vi "View one AI param.vi"(5 "ActivateAIView":bool, 7 "conninfo":T4={"host"="localhost", "port"="5432", "client_encoding"="WIN1251", "dbname"="system", "user"="postgres", "password"=""}, 9 "AIP":T2, 10 "AI_State":T1[](array[typedef]), 11 "AITable":dbl[](array[numeric]) format="%#.0f") -> (0 "error out":errorcluster)   [LabVIEW 2019, in "Inputs.lvlib"]
uses:
  Inputs.lvlib
  Database/ctl/Coninfo.ctl
  Ctl/AI.ctl
  Ctl/AI short.ctl
  Ctl/Parameter State.ctl
  Ctl/AIParamColumns.ctl
  Database/PostgreSQL2LabVIEW/libpqUtility64/src/PQexecute.vi
  Database/PostgreSQL2LabVIEW/libpqUtility64/src/PQconnect.vi
  Database/PostgreSQL2LabVIEW/libpqUtility64/src/PQclose.vi
  Database/PostgreSQL2LabVIEW/libpqlv64/src/PQresultErrorMessage.vi
  Database/PostgreSQL2LabVIEW/libpqUtility64/src/PQclear.vi
  Database/PostgreSQL2LabVIEW/libpqlv64/src/PQsendQuery.vi
  Database/PostgreSQL2LabVIEW/libpqlv64/src/PQgetResult.vi
  Database/PostgreSQL2LabVIEW/libpqlv64/src/PQresultStatus.vi
  Database/PostgreSQL2LabVIEW/libpqlv64/src/PQfinish.vi
  Database/PostgreSQL2LabVIEW/libpqlv64/src/PQconnectdb.vi
  Database/PostgreSQL2LabVIEW/libpqlv64/src/PQerrorMessage.vi
  Database/PostgreSQL2LabVIEW/libpqlv64/src/PQstatus.vi
  Database/PostgreSQL2LabVIEW/libpqlv64/src/PQclear.vi
  Database/PostgreSQL.lvlib
panel:
  in  "instrument_min_offset":dbl min=-32768.0 max=65535.0 step=1.0 format="%#.0f"
  in  "time_const":dbl min=-32768.0 max=65535.0 step=1.0 format="%#.0f"
  in  "instrument_offset":dbl min=-32768.0 max=65535.0 step=1.0 format="%#.0f"
  in  "instrument_gain":dbl min=-32768.0 max=65535.0 step=1.0 format="%#.0f"
  out "fcode_full":string="кгс/см2"
  out "AI_1":dbl format="%#.1f"
  in  "Param":i32[](listbox) caption="Параметры"
  in  "fcodef":string
  in  "fcode":string
  in  "d":dbl min=-32768.0 max=65535.0 step=1.0 format="%#.0f"
  in  "instrument_max_offset":dbl min=-32768.0 max=65535.0 step=1.0 format="%#.0f"
  in  "input_pv_max":dbl format="%#.1f"
  in  "input_pv_min":dbl format="%#.1f"
  in  "input_register_max":dbl min=-32768.0 max=65535.0 step=1.0 format="%#.0f"
  in  "input_register_min":dbl min=-32768.0 max=65535.0 step=1.0 format="%#.0f"
  out "units":string="кгс/см2"
  in  "instrument_range_max":dbl format="%#.1f"
  in  "process_range_max":dbl format="%#.1f"
  in  "process_high_acd":dbl format="%#.1f"
  in  "process_high_alr":dbl format="%#.1f"
  in  "process_low_alr":dbl format="%#.1f"
  in  "process_low_acd":dbl format="%#.1f"
  in  "process_range_min":dbl format="%#.1f"
  in  "instrument_range_min":dbl format="%#.1f"
  # "Настройка пределов"
  # "верхнийний предел датчика"
  # "верхний предел достоверных показаний"
  # "верхний аварийный предел"
  # "верхний предупредительный предел"
  # "нижний предупредительный предел"
  # "нижний аварийный предел"
  # "нижний предел достоверных показаний"
  # "нижний предел датчика"
  # "Настройка датчика"
  # "Y"
  # "значение сигнала максимум (Ymax)"
  # "значение сигнала минимум (Ymin)"
  # "X"
  # "входной регистр минимум (Xmin)"
  # "входной регистр максимум (Xmax)"
  # "Analog parameters"
  # "Description of analog parameters"
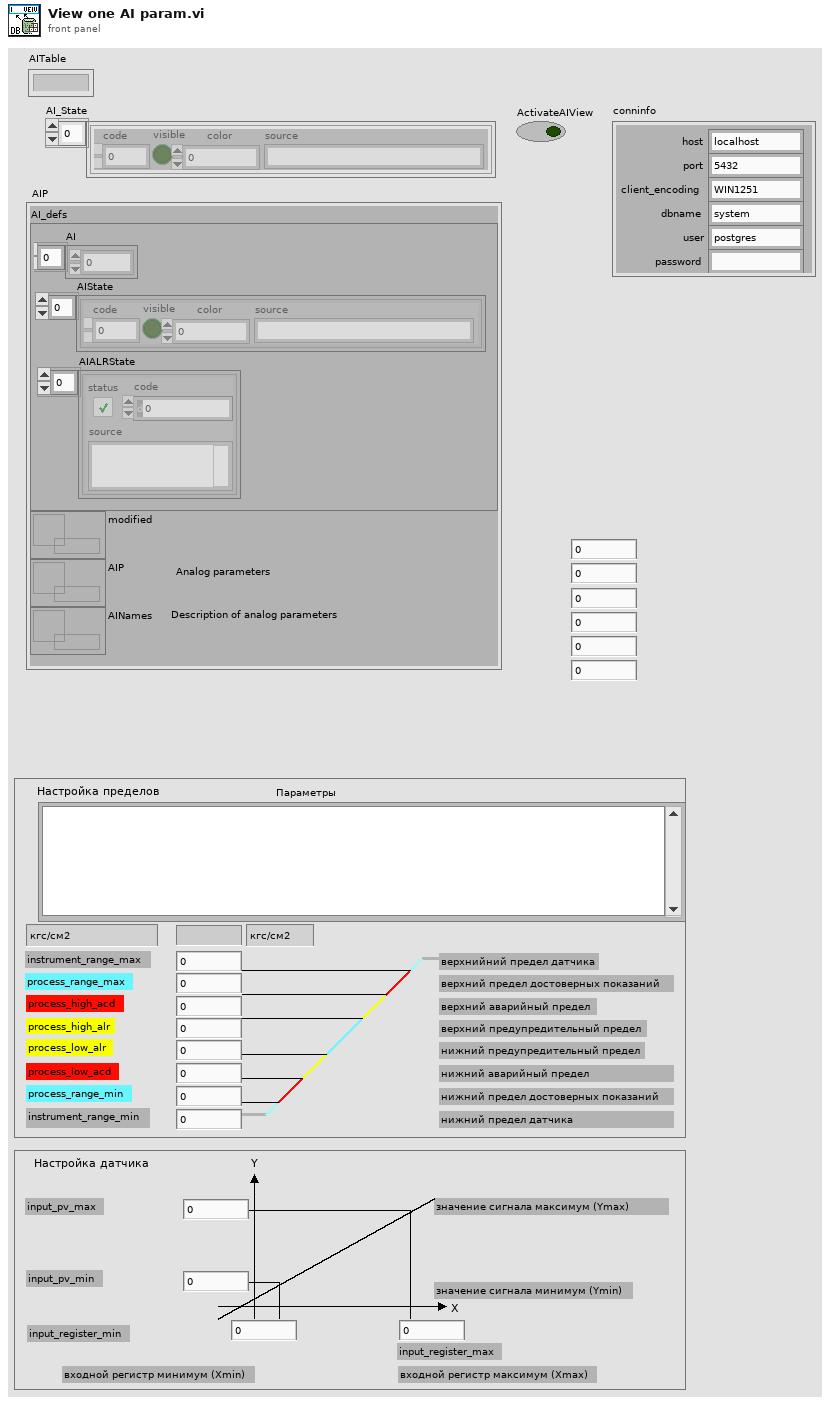
[diagram p1: front panel]
types:
  T1 = typedef "Inputs.lvlib/Parameter State.ctl" = cluster{"code":i32, "visible":bool, "color":u32, "source":string}
  T2 = typedef "Inputs.lvlib/AI.ctl" = cluster{"AI_defs":T3, "modified":refnum<data-value>, "AIP":refnum<data-value>, "AINames":refnum<data-value>}
  T3 = typedef "Inputs.lvlib/AI short.ctl" = cluster{"AI":dbl[], "AIState":T1[], "AIALRState":errorcluster[]}
  T4 = typedef "PostgreSQL.lvlib/Coninfo.ctl" = cluster{"host":string, "port":string, "client_encoding":string, "dbname":string, "user":string, "password":string}
  T5 = enum32{"Invalid", "Standard", "Closed", "Hidden", "Minimized", "Maximized"}
  T6 = typedef "Inputs.lvlib/AIParamColumns.ctl" = enum16{"instrument_gain", "instrument_offset", "time_const", "instrument_min_offset", "instrument_range_min", "process_range_min", "process_low_acd", "process_low_alr", "process_high_alr", "process_high_acd", "process_range_max", "instrument_range_max", "instrument_max_offset", "d", "input_register_min", "input_register_max", "input_pv_min", "input_pv_max", "module_fcode_full", "control_channel_num", "ip_adress", "fcode", "fcodef", "fcode_full", "fname", "process_units"}
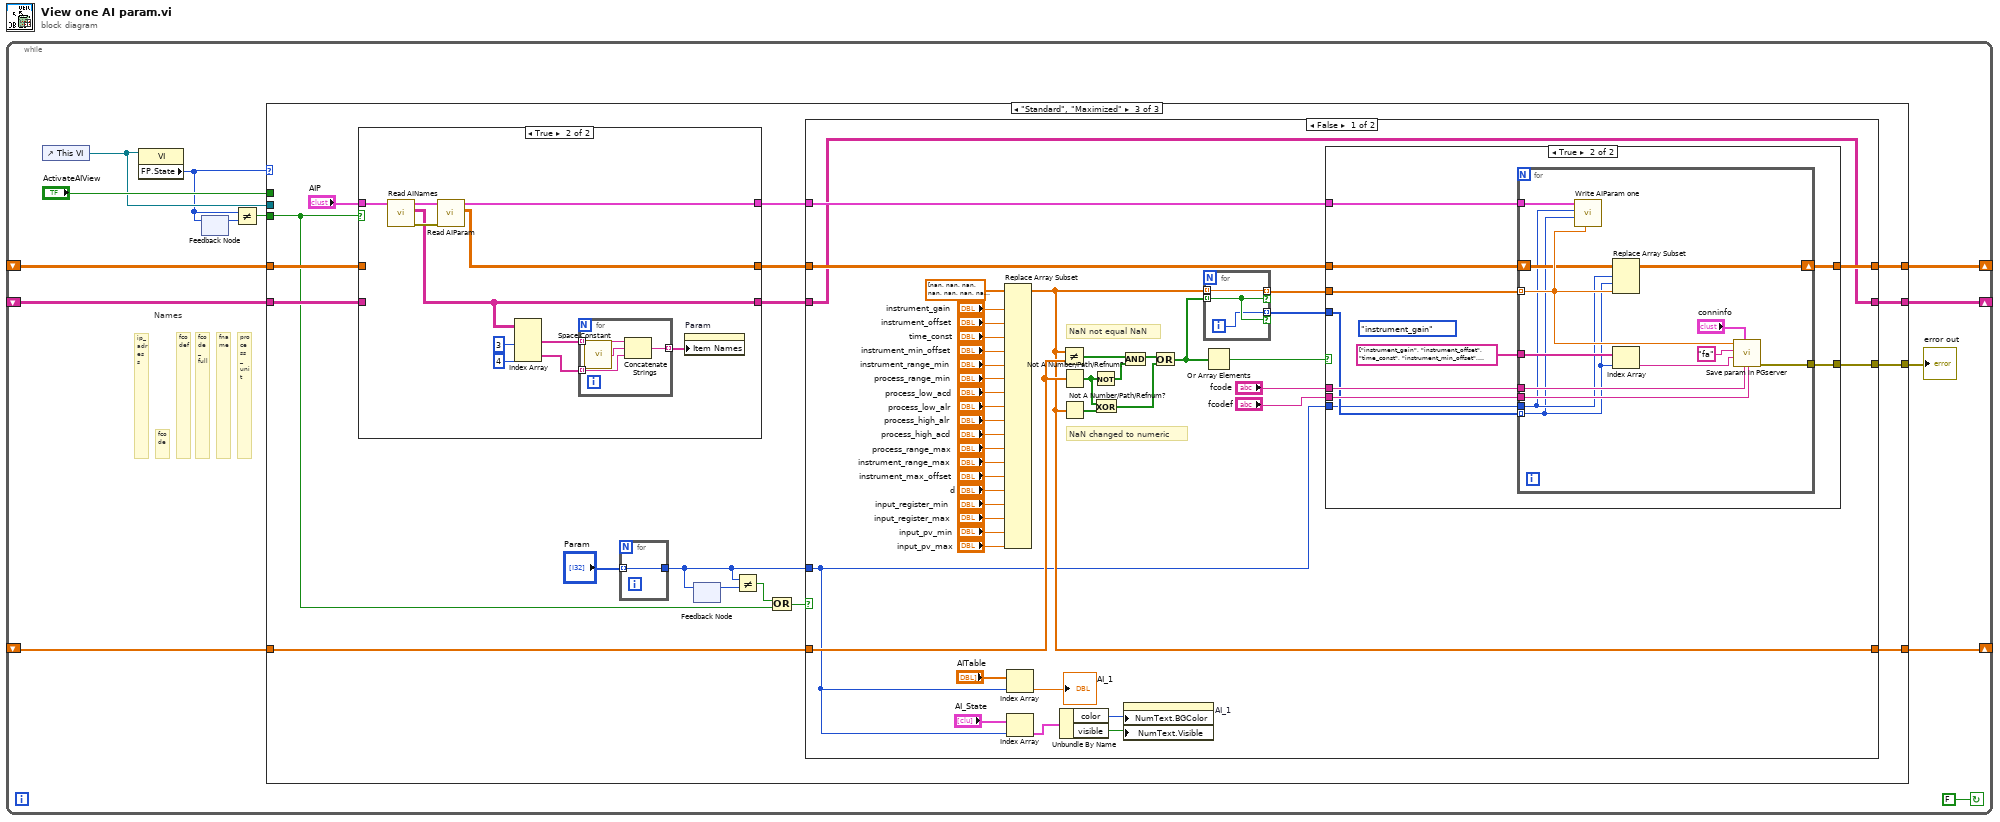
[diagram p0: block diagram]
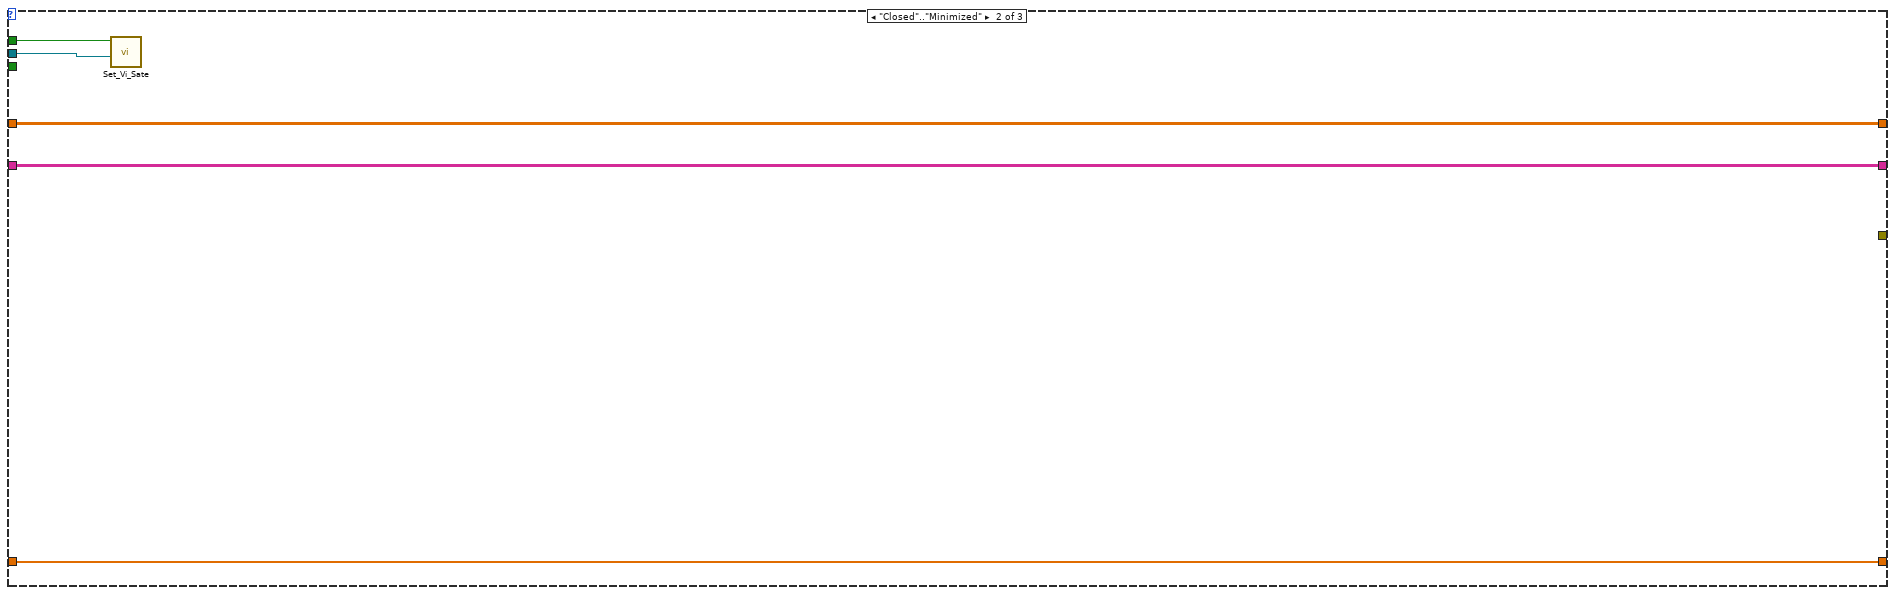
[diagram p3: hidden frame]
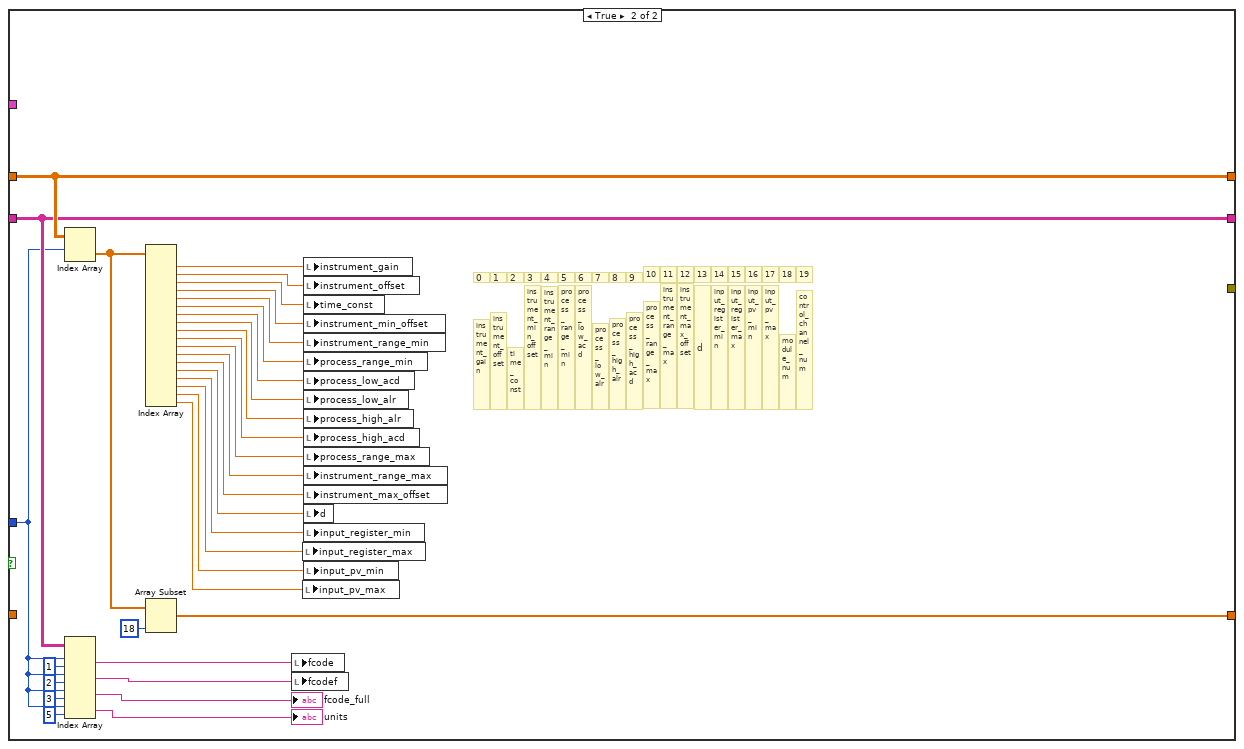
[diagram p6: hidden frame]
diagram:
  n1 = while {
    shift-right: [w6] -> _
    shift-left: _ -> [w4]
    shift-right: [w5] -> _
    shift-left: _ -> [w3]
    shift-right: [w2] -> _
    shift-left: _ -> [w1]
    stop <- FALSE continue-if-true
    # "fcodef"
    # "ip_adress"
    # "process_unit"
    # "fname"
    # "fcode_full"
    # "fcode"
    # "Names"
    n2 = control-ref of="This VI"() -> (w12:refnum<vi>)
    n3 = property class="VI"(reference=w12) -> ("FP.State"=w9:T5)  [unwired: 1 in, 2 out]
    n4 = feedback #1() -> (w10:T5)  [unwired: 1 in]
    n5 = feedback-in #1(w9) -> ()
    n6 = Not Equal?(x=w9, y=w10) -> (x != y?=w8:bool)
    n7 = case shown="\"Standard\", \"Maximized\"" w9 {
      tunnel: "ActivateAIView" -> [_ w21 _]
      tunnel: w12 -> [_ w20 _]
      tunnel: [_ _ w28] -> w11
      tunnel: w8 -> [_ _ w30]
      tunnel: [w16 w19 w22] -> w6
      tunnel: [w15 w18 w24] -> w5
      tunnel: w4 -> [w16 w19 w32]
      tunnel: w3 -> [w15 w18 w31]
      tunnel: [w14 w17 w27] -> w2
      tunnel: w1 -> [w14 w17 w26]
      frame "Invalid", Default {
      }
      frame "Closed".."Minimized" {
        n8 = call "Set_Vi_Sate.vi"("VI"=w20, "Activate (F)"=w21) -> ()  [unwired: 9 in, 1 out]
      }
      frame "Standard", "Maximized" {
        n9 = case shown="True" w30 {
          tunnel: [w41 w45] -> w25
          tunnel: [w42 w44] -> w33
          tunnel: "AIP" -> [w40 w46]
          tunnel: w32 -> [w42 _]
          tunnel: w31 -> [w41 _]
          tunnel: [w40 w43] -> w23
          frame False {
          }
          frame True {
            n10 = call "Read AINames.vi"("AI in"=w46) -> ("error out"=w48:errorcluster, "AINames"=w45:string[][], "AI out"=w47:T2)  [unwired: 8 in]
            n11 = call "Read AIParam.vi"("error in (no error)"=w48, "AI in"=w47) -> ("AIParam"=w44:dbl[][], "AI out"=w43:T2)  [unwired: 7 in, 1 out]
            n12 = Index Array(array=w45, index (col) #1=3 ("index (row)"), index (col) #2=4 ("index (row)")) -> (element #1=w52:string[], element #2=w50:string[])  [unwired: 2 in]
            n13 = for {
              tunnel: w52 -> [w57] mode=indexing
              tunnel: w50 -> [w55] mode=indexing
              tunnel: [w54] -> w49 mode=indexing
              n14 = call <vilib>:"Space Constant.vi"() -> ("String"=w56:string)
              n15 = Concatenate Strings(w57, w56, w55) -> (w54:string)
            }
            n16 = property on="Param" class="LstBox (strict)"("Item Names"=w49) -> ()  [unwired: 2 in, 2 out]
          }
        }
        n17 = for {
          tunnel: "Param" -> [w39] mode=indexing
          tunnel: [w39] -> w29
        }
        n18 = feedback #2() -> (w38:i32)  [unwired: 1 in]
        n19 = feedback-in #2(w29) -> ()
        n20 = Not Equal?(x=w29, y=w38) -> (x != y?=w36:bool)
        n21 = Or(x=w36, y=w30) -> (x .or. y?=w37:bool)
        n22 = case shown="False" w37 {
          tunnel: w29 -> [w63 w136]
          tunnel: w25 -> [w64 w141]
          tunnel: w33 -> [w82 w142]
          tunnel: [w85 _] -> w28
          tunnel: [w70 w140] -> w27
          tunnel: w26 -> [w73 _]
          tunnel: [w74 w142] -> w22
          tunnel: [w64 w141] -> w24
          tunnel: w23 -> [w81 _]
          frame False {
            # "NaN changed to numeric"
            # "NaN not equal NaN"
            n23 = Replace Array Subset(array=dbl[] [nan, nan, nan, nan, nan, nan, nan, nan, nan, nan, nan, nan, nan, nan, nan, nan, nan, nan] ("Parameters table"), new element #1="instrument_gain", new element #2="instrument_offset", new element #3="time_const", new element #4="instrument_min_offset", new element #5="instrument_range_min", new element #6="process_range_min", new element #7="process_low_acd", new element #8="process_low_alr", new element #9="process_high_alr", new element #10="process_high_acd", new element #11="process_range_max", new element #12="instrument_range_max", new element #13="instrument_max_offset", new element #14="d", new element #15="input_register_min", new element #16="input_register_max", new element #17="input_pv_min", new element #18="input_pv_max") -> (w70:dbl[])  [unwired: 18 in]
            n24 = Index Array(array="AITable", index=w63) -> (element=→"AI_1":dbl)
            n25 = Index Array(array="AI_State", index=w63) -> (element=w77:T1)
            n26 = Unbundle By Name(w77) -> ("color"=w76:u32, "visible"=w75:bool)
            n27 = Not Equal?(x=w70, y=w73) -> (x != y?=w71:bool[])
            n28 = Not A Number/Path/Refnum?(number/path/refnum=w73) -> (NaN/Path/Refnum?=w66:bool[])
            n29 = Not A Number/Path/Refnum?(number/path/refnum=w70) -> (NaN/Path/Refnum?=w65:bool[])
            n30 = Not(x=w66) -> (.not. x?=w67:bool[])
            n31 = Exclusive Or(1:w65, 2:w66) -> (0:w69:bool[])
            n32 = And(x=w71, y=w67) -> (x .and. y?=w68:bool[])
            n33 = property on="AI_1" class="DigNum (strict)"("NumText.BGColor"=w76, "NumText.Visible"=w75) -> ()  [unwired: 2 in, 2 out]
            n34 = Or(x=w68, y=w69) -> (x .or. y?=w72:bool[])
            n35 = for {
              tunnel: w70 -> [w105] mode=indexing
              tunnel: w72 -> [w104] mode=indexing
              tunnel: [w105] -> w84 mode=indexing if=w104
              tunnel: [w103] -> w58 mode=indexing if=w104
              i -> [w103]
            }
            n36 = Or Array Elements(Boolean array=w72) -> (logical OR=w83:bool)
            n37 = case shown="True" w83 {
              tunnel: "fcode" -> [_ w116]
              tunnel: [_ w115] -> w85
              tunnel: w63 -> [_ w111]
              tunnel: "fcodef" -> [_ w114]
              tunnel: w84 -> [_ w112]
              tunnel: w58 -> [_ w113]
              tunnel: w82 -> [w106 w110]
              tunnel: w81 -> [_ w108]
              tunnel: [w106 w109] -> w74
              frame False {
              }
              frame True {
                (unwired) AIParamColumns."instrument_gain" ("AIParamColumns")
                n38 = for {
                  tunnel: w116 -> [w128]
                  tunnel: [w125] -> w115
                  tunnel: w111 -> [w120]
                  tunnel: w114 -> [w127]
                  tunnel: string[] ["instrument_gain", "instrument_offset", "time_const", "instrument_min_offset", "instrument_range_min", "process_range_min", "process_low_acd", "process_low_alr", "process_high_alr", "process_high_acd", "process_range_max", "instrument_range_max", "instrument_max_offset", "d", "input_register_min", "input_register_max", "input_pv_min", "input_pv_max", "module_fcode_full", "control_channel_num", "ip_adress", "fcode", "fcodef", "fcode_full", "fname", "process_units"] ("AIParamColumns") -> [w124]
                  tunnel: w113 -> [w119] mode=indexing
                  tunnel: w112 -> [w129] mode=indexing
                  shift-right: [w122] -> w109
                  shift-left: w110 -> [w123]
                  tunnel: w108 -> [w121]
                  n39 = call "Write AIParam one.vi"("AIParam"=w129, "Param column"=w119, "Param number"=w120, "AI in"=w121) -> ()  [unwired: 6 in, 2 out]
                  n40 = Replace Array Subset(array=w123, new element=w129, index (row)=w120, index (col)=w119) -> (w122:dbl[][])
                  n41 = Index Array(array=w124, index=w119) -> (element=w126:string)
                  n42 = call "Save param in PGserver.vi"("Param row name 2"=w127, "Param row name1"=w128, "conninfo"="conninfo", "Param column Name"=w126, "Param Table"="fa", "Parameter"=w129) -> ("error out"=w125:errorcluster)  [unwired: 5 in]
                }
              }
            }
          }
          frame True {
            # "control_channel_num"
            # "module_num"
            # "input_pv_max"
            # "input_pv_min"
            # "input_register_max"
            # "input_register_min"
            # "d"
            # "instrument_max_offset"
            # "instrument_range_max"
            # "process_range_max"
            # "process_high_acd"
            # "process_high_alr"
            # "process_low_alr"
            # "process_low_acd"
            # "process_range_min"
            # "instrument_range_min"
            # "instrument_min_offset"
            # "time_const"
            # "instrument_gain"
            # "instrument_offset"
            # "19"
            # "18"
            # "17"
            # "16"
            # "15"
            # "14"
            # "13"
            # "12"
            # "11"
            # "10"
            # "9"
            # "8"
            # "7"
            # "6"
            # "5"
            # "4"
            # "3"
            # "2"
            # "0"
            # "1"
            n43 = Index Array(array=w142, index (row)=w136) -> (element=w144:dbl[])  [unwired: 1 in]
            n44 = Index Array(array=w141, index (row) #1=w136, index (col) #1=1 ("length"), index (row) #2=w136, index (col) #2=2 ("length"), index (row) #3=w136, index (col) #3=3 ("length"), index (row) #4=w136, index (col) #4=5 ("length")) -> (element #1=w139:string, element #2=w138:string, element #3=→"fcode_full":string, element #4=→"units":string)
            n45 = Index Array(array=w144) -> (element #1=w130:dbl, element #2=w131:dbl, element #3=w132:dbl, element #4=w133:dbl, element #5=w158:dbl, element #6=w157:dbl, element #7=w156:dbl, element #8=w155:dbl, element #9=w154:dbl, element #10=w153:dbl, element #11=w152:dbl, element #12=w151:dbl, element #13=w146:dbl, element #14=w145:dbl, element #15=w150:dbl, element #16=w149:dbl, element #17=w148:dbl, element #18=w147:dbl)  [unwired: 18 in]
            n46 = Array Subset(array=w144, length=18) -> (w140:dbl[])  [unwired: 1 in]
            n47 = local write "fcode"(w139) -> ()
            n48 = local write "fcodef"(w138) -> ()
            n49 = local write "input_register_max"(w149) -> ()
            n50 = local write "input_pv_max"(w147) -> ()
            n51 = local write "instrument_gain"(w130) -> ()
            n52 = local write "instrument_offset"(w131) -> ()
            n53 = local write "time_const"(w132) -> ()
            n54 = local write "instrument_min_offset"(w133) -> ()
            n55 = local write "instrument_range_min"(w158) -> ()
            n56 = local write "process_range_min"(w157) -> ()
            n57 = local write "process_low_acd"(w156) -> ()
            n58 = local write "process_low_alr"(w155) -> ()
            n59 = local write "process_high_alr"(w154) -> ()
            n60 = local write "process_high_acd"(w153) -> ()
            n61 = local write "process_range_max"(w152) -> ()
            n62 = local write "instrument_range_max"(w151) -> ()
            n63 = local write "instrument_max_offset"(w146) -> ()
            n64 = local write "d"(w145) -> ()
            n65 = local write "input_register_min"(w150) -> ()
            n66 = local write "input_pv_min"(w148) -> ()
          }
        }
      }
    }
    "error out" <- w11
  }
